vi "N-Parametric Double FFT Mesurament Test SLOW (con Sottrazione Fondo).vi"() -> ()   [LabVIEW 2014]
uses:
  <vilib>/Platform/TimedLoop/XDataNode/timing_clust.ctl
  <vilib>/Platform/TimedLoop/XDataNode/nitl_modes.ctl
  <vilib>/Platform/TimedLoop/XDataNode/wakeup.ctl
  <vilib>/rvi/Analysis/measure/FFT/simModelSupport/niFPGA FFT Streaming Sim Properties.ctl
  <vilib>/rvi/Analysis/measure/FFT/simModelSupport/niFPGA FFT Sim Stream Group Properties.ctl
  <vilib>/rvi/Analysis/measure/FFT/simModelSupport/niFPGA FFT Sim Types.ctl
  <vilib>/rvi/Analysis/measure/FFT/simModelSupport/niFpgaFFTSimArithmeticProperties.ctl
  <vilib>/rvi/Analysis/measure/FFT/simModelSupport/niFpgaFFTSimDfxp.ctl
  <vilib>/fxp/LVFixedPointQuantizationPolicyTypeDef.ctl
  <vilib>/rvi/Analysis/measure/FFT/XNode/niFpgaFFTButterflyDelays.ctl
  <vilib>/rvi/Emulation/niFpgaSctlEmulationGetInTimedLoop.vi
  <vilib>/rvi/Emulation/niFpgaEmulationReportErrorSimple.vi
  <vilib>/rvi/Emulation/niFpgaGetClockAttributes.vi
  <vilib>/rvi/Emulation/niFpgaCriticalErrorInLSC.vi
  <vilib>/rvi/Emulation/niFpgaEmulationIsFPGAContextNoSignature.vi
  <vilib>/rvi/DataTransferAndStorage/Container/Common/niFpgaContainerGetUniqueNameForEmu.vi
  <vilib>/rvi/Memory/Memory_Emulation/niFpgaMemoryEmulationCacheClearOnFirstRun.vi
  <vilib>/rvi/Memory/Memory_Emulation/nirvimemoryEmulationManagerCache_MakeExclusive.vi
  <vilib>/rvi/Memory/Memory_Emulation/niFpgaMemoryEmulationValidateCache.vi
  <vilib>/rvi/Memory/Memory_Emulation/nirvimemoryEmulationManagerCache_InsertValue.vi
  <vilib>/Utility/error.llb/Clear Errors.vi
  <vilib>/rvi/Memory/Memory_Emulation/nirvimemoryEmulationManagerCache_ReleaseExclusive.vi
  <vilib>/rvi/Memory/Memory_Emulation/nirvimemoryEmulationManagerCache_GetValue.vi
  <vilib>/rvi/Memory/Memory_Emulation/nirvimemoryEmulationManagerCache_SetValue.vi
  <vilib>/rvi/Emulation/niFpgaProcessEmulError.vi
  <vilib>/rvi/errors/niFpgaSetErrorForExecOnDevCompSimple.vi
  <vilib>/rvi/eio/common/nirviEmuReportErrorAndStop.vi
  <vilib>/rvi/FIFO/Fifo_Resource/nirvififoEmulationSetSize.vi
  <vilib>/rvi/FIFO/Fifo_Resource/nirviFifoEmulationQueueMgr.vi
  <instcachedir>/0/nirviFifoEmulationQueueMgr_E5CAEC123FF24DC58D834DCA3CDAA9B5.lvgen/nirviFifoEmulationQueueMgr_E5CAEC123FF24DC58D834DCA3CDAA9B5_010.vi
  <vilib>/rvi/FIFO/Fifo_Resource/nirvififoEmulationCreateLock.vi
  <vilib>/rvi/FIFO/Fifo_Resource/nirvififoEmulationObtainLock.vi
  <vilib>/rvi/FIFO/Fifo_Resource/nirvififoEmulationReleaseLock.vi
  <vilib>/rvi/occurrence/nirviWaitOnOccurrenceBase.vi
  <vilib>/rvi/errors/nirviReportUnexpectedCaseInternalError.vi
  <vilib>/rvi/errors/nirviReportUnexpectedCaseInternalError (U32).vi
  <vilib>/rvi/FIFO/Fifo_Resource/nirvififoEmulationDetermineInputValidOut.vi
  <vilib>/rvi/Memory/Memory_Emulation/nirvimemoryFastEmulation.vi
  <vilib>/rvi/Memory/Memory_Emulation/nirvimemoryEmulation.vi
  <vilib>/rvi/eio/common/nirviEmuTemplateMethod_errors.vi
  <vilib>/rvi/Analysis/measure/FFT/simModelSupport/niFpgaFFTSimModelStreamingCore.vi
  <vilib>/rvi/interface/RandomDataEmulation/niFpgaRandomDataHandleErrors.vi
  <vilib>/Platform/TimedLoop/XDataNode/XDataNode.xnode
  <vilib>/rvi/DataTransferAndStorage/Container/XNode/niFpgaContainer.xnode
  <vilib>/rvi/DataTransferAndStorage/Register/Emulation/niFpgaRegisterEmulation.vi
  <vilib>/rvi/FIFO/Fifo_Resource/nirvififoEmulationRead.vi
  <vilib>/rvi/FIFO/Fifo_Resource/nirvififoEmulationWrite.vi
  <vilib>/eio/EIOMethodNode/EIOMethodNode.xnode
  <vilib>/rvi/Analysis/measure/FFT/XNode/niFpgaFFT.xnode
  <vilib>/rvi/interface/RandomDataEmulation/nirviRandomDataFpgaReadWriteTemplate.vi
  <vilib>/Platform/TimedLoop/XDataNode/XDNodeRunTimeDep.lvlib
panel:
  in  "n-bit (2^nbit medie)":i32=8
  in  "n":u32=1
  in  "Latency points":u32
  in  "snapshot":bool
  in  "lower limit 2":u32=682
  in  "lower limit 1":u32=57
  in  "upper limit 2":u32=1193
  in  "upper limit 1":u32=568
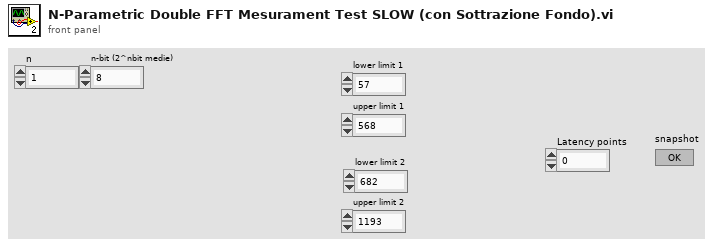
[diagram p1: front panel]
types:
  T1 = typedef "XDNodeRunTimeDep.lvlib/timing_clust.ctl" = cluster{"Expected End [f-1]":u64, "Actual End [f-1]":u64, "Finished Late? [f-1]":bool, "Expected End [i-1]":u64, "Actual End [i-1]":u64, "Finished Late? [i-1]":bool, "Expected Start [i]":u64, "Actual Start [i]":u64, "Expected Start [f]":u64, "Actual Start [f]":u64, "Source Name":string, "Structure Name":string, "Period":i64, "Deadline":i64, "Offset":i64, "Start":i64, "Priority":i32, "Timeout":i32, "Mode":T2, "Wakeup Reason":T3, "Error":errorcluster, "Source Type":string, "Secondary Source Type":string, "Global End Time":u64, "Global Start Time":u64, "Frame Duration":u64, "Iteration Duration":u64, "Assigned CPU":i32, "I/O Scan Engine Mode":u32}
  T2 = typedef "XDNodeRunTimeDep.lvlib/nitl_modes.ctl" = enum32{"No Change", "Process missed periods, maintain original phase", "Discard missed periods, maintain original phase", "Process missed periods, ignore original phase", "Discard missed periods, ignore original phase"}
  T3 = typedef "XDNodeRunTimeDep.lvlib/wakeup.ctl" = enum32{"Normal", "Aborted", "Asynchronous wakeup", "Timing source error", "Timed loop error", "Timeout"}
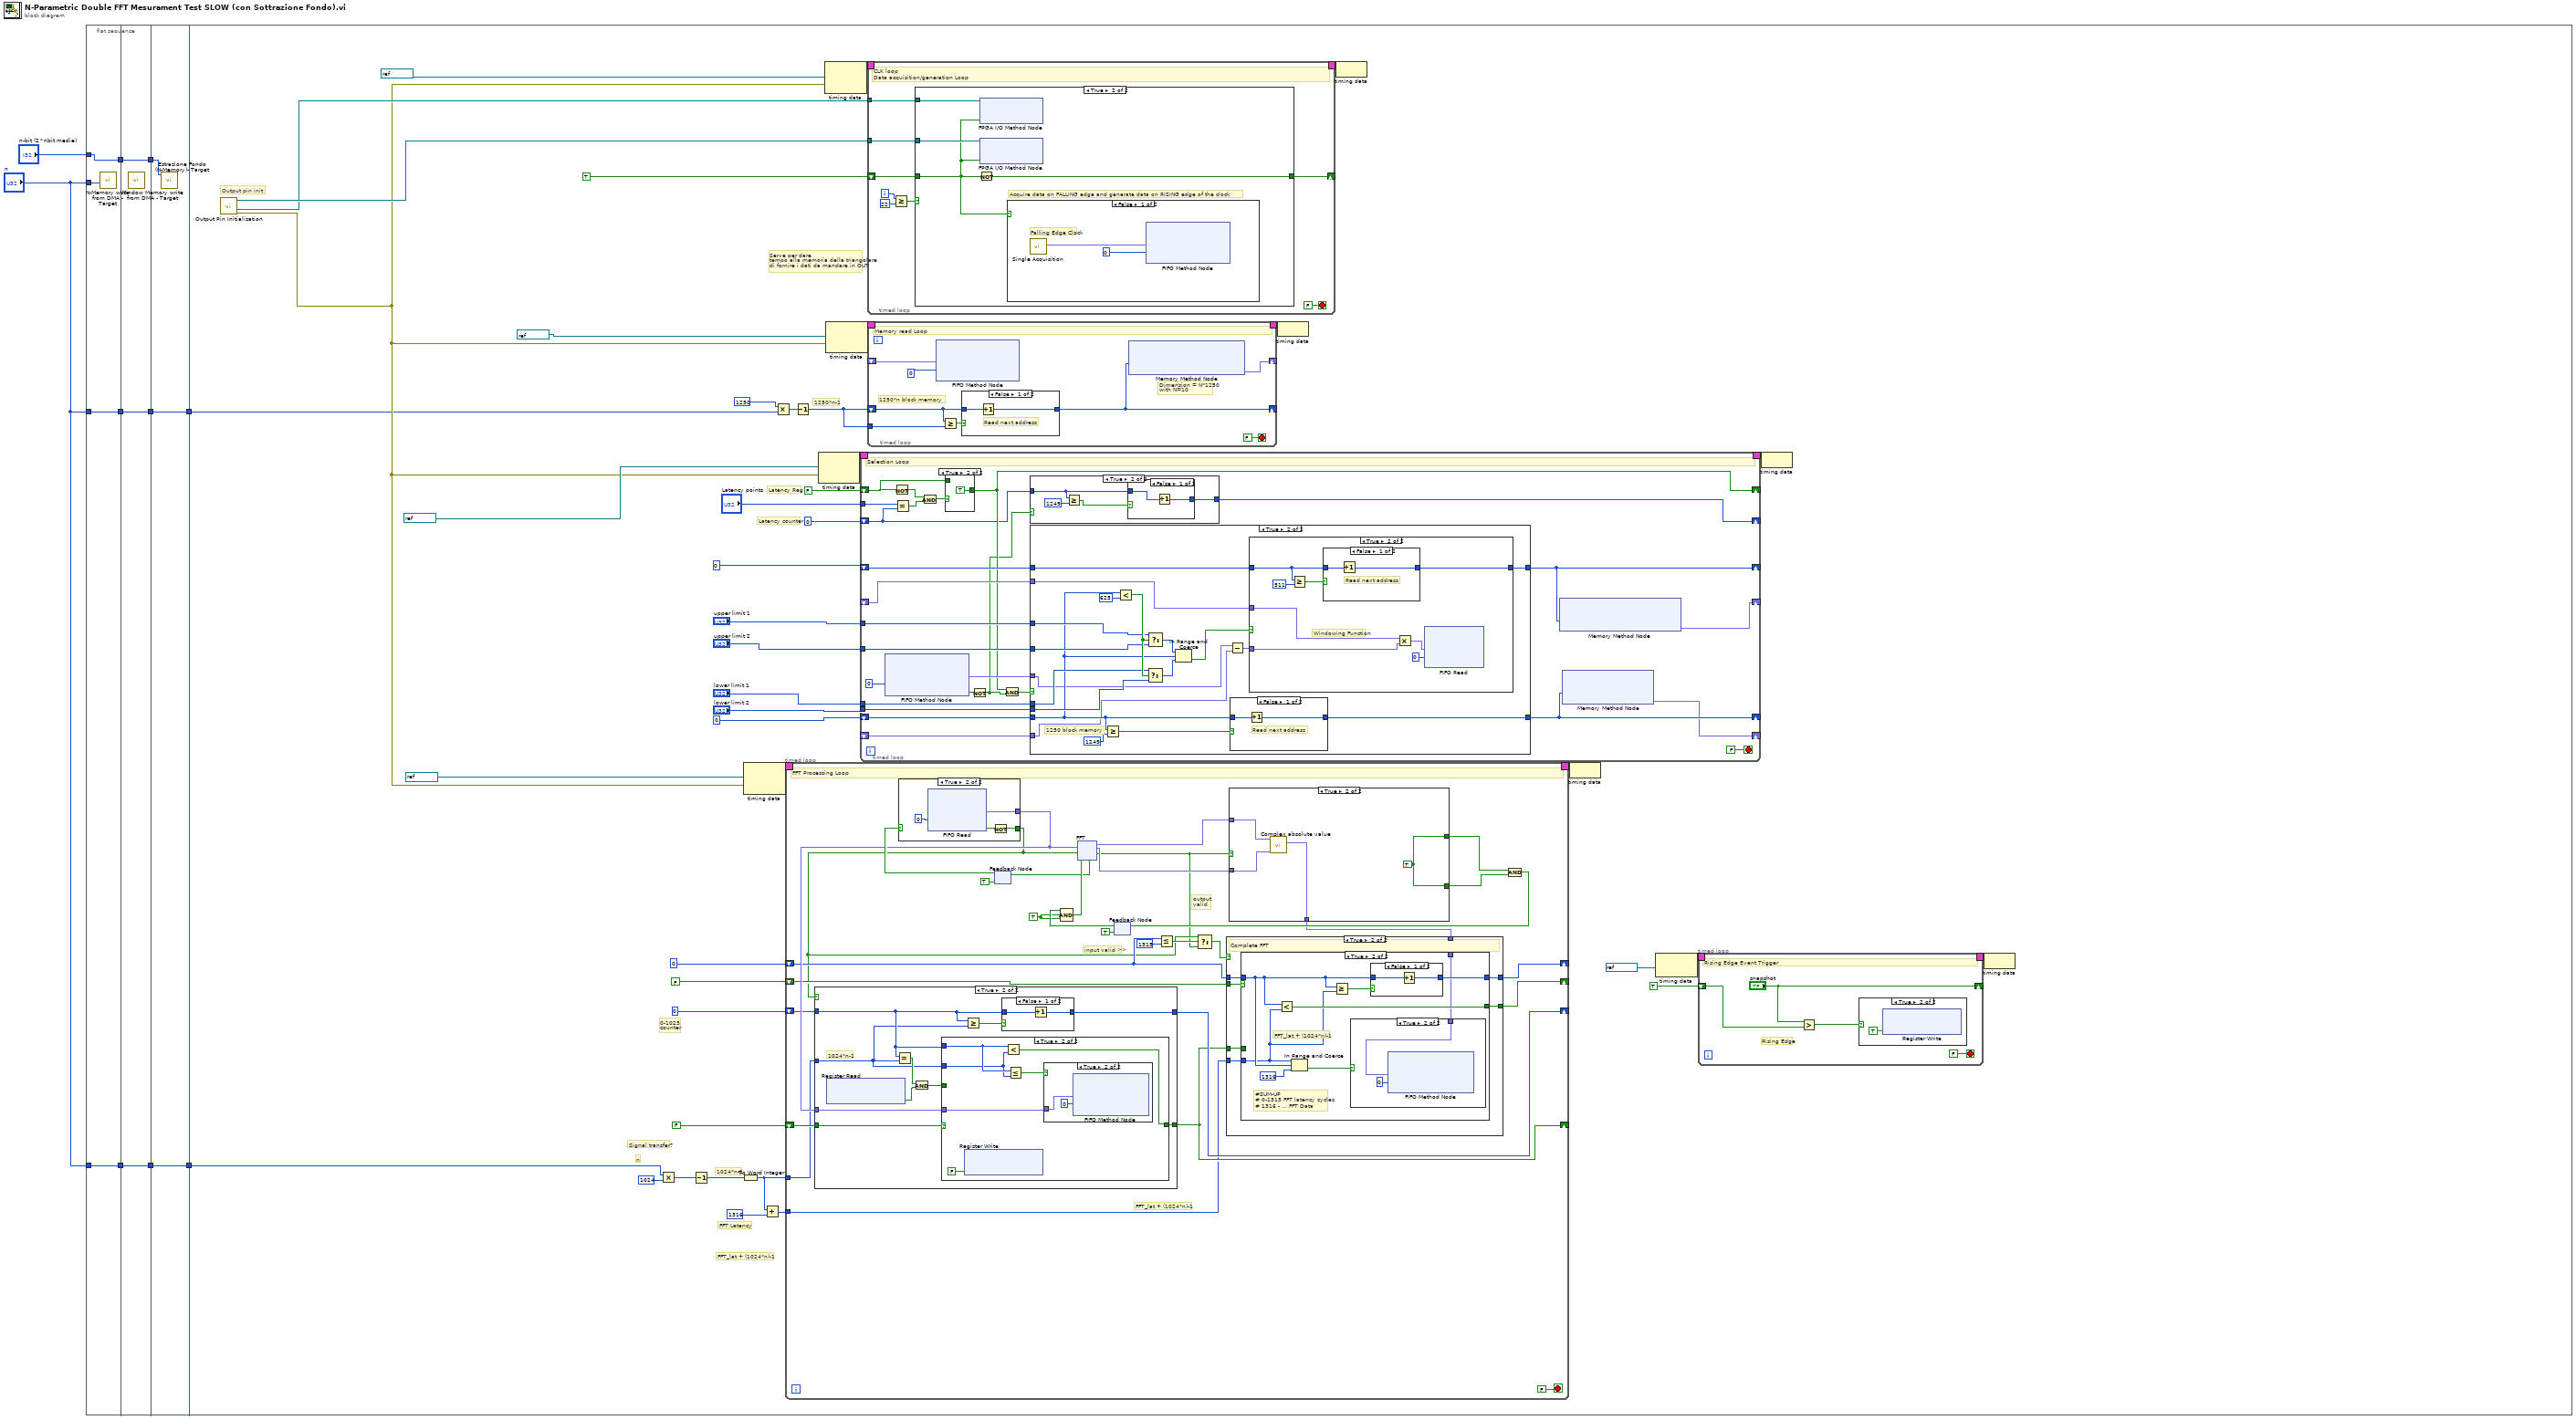
[diagram p0: block diagram]
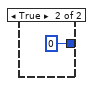
[diagram p4: hidden frame]
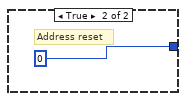
[diagram p8: hidden frame]
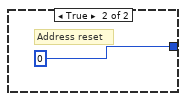
[diagram p9: hidden frame]
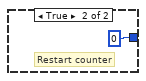
[diagram p13: hidden frame]
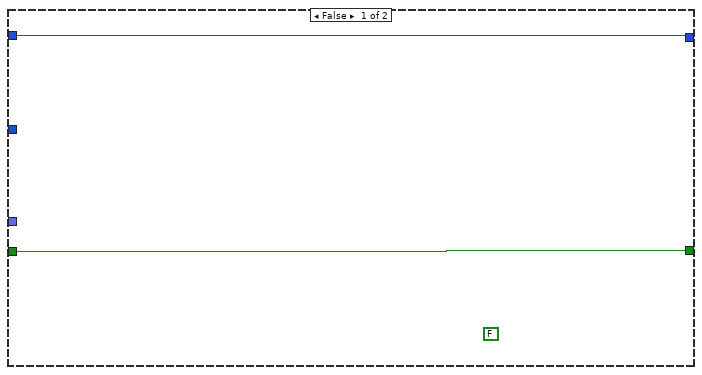
[diagram p14: hidden frame]
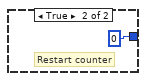
[diagram p17: hidden frame]
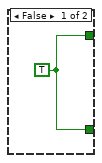
[diagram p18: hidden frame]
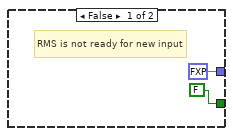
[diagram p19: hidden frame]
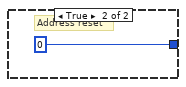
[diagram p20: hidden frame]
diagram:
  n1 = flat-sequence {
    tunnel: "n" -> [w14]
    tunnel: [w13] -> w10
    tunnel: "n" -> [w13]
    tunnel: "n" -> [w12]
    tunnel: [w12] -> w8
    tunnel: [w11] -> w3
    tunnel: "n-bit (2^nbit medie)" -> [w11]
    tunnel: w10 -> [w17]
    tunnel: [w17] -> w7
    tunnel: w8 -> [w16]
    tunnel: [w16] -> w5
    tunnel: w3 -> [w15]
    tunnel: [w15] -> w2
    tunnel: w7 -> [w20]
    tunnel: [w20] -> w6
    tunnel: w5 -> [w19]
    tunnel: [w19] -> w4
    tunnel: w2 -> [w18]
    tunnel: w6 -> [w30]
    tunnel: w4 -> [w21]
    frame #0 {
      n2 = call "N-Memory write from DMA - Target.vi"("n"=w14) -> ()  [unwired: 11 in]
    }
    frame #1 {
      n3 = call "Window Memory write from DMA - Target.vi"() -> ()  [unwired: 12 in]
    }
    frame #2 {
      n4 = call "Estrazione Fondo (N-Memory)- Target.vi"("n-bit (2^nbit medie)"=w18) -> ()  [unwired: 11 in]
    }
    frame #3 {
      # "1250*n-1"
      # "FFT_lat + (1024*n)-1"
      # "FFT Latency"
      # "n"
      # "1024*n-1"
      # "Serve per dare\ntempo alla memoria della triangolare\ndi fornire i dati da mandare in OUT"
      # "Latency counter"
      # "Latency Reg"
      # "0-1023\ncounter"
      # "Signal transfer?"
      # "Output pin init"
      n5 = call "Output Pin Initialization.vi"() -> ("error out"=w48:errorcluster, "I/O Out Clock DAC (pin16)"=w52:refnum<k21>, "I/O Out Clock ADC (pin17)"=w53:refnum<k21>)  [unwired: 8 in]
      n6 = Multiply(x=w30, y=u32 1024) -> (x*y=w31:u32)
      n7 = Decrement(x=w31) -> (x-1=w29:u32)
      n8 = To Word Integer(number=w29) -> (16bit integer=w27:i16)
      n9 = node-c288(refnum<k21> "30MHz" ("Source Name"), w48) -> (w60:T1)
      n10 = Add(x=w27, y=i16 1316) -> (x+y=w25:i16)
      n11 = Multiply(x=u32 1250, y=w21) -> (x*y=w23:u32)
      n12 = timed-loop {
        timing: w60 -> [_]
        timing-out: [_] -> w59
        shift-right: [w168] -> _
        shift-left: FALSE -> [w171]
        shift-right: [w172] -> _
        shift-left: i16 0 -> [w169]
        shift-right: [w167] -> _
        shift-left: FALSE -> [w166]
        shift-right: [w165] -> _
        shift-left: i16 0 -> [w163]
        tunnel: w27 -> [w156]
        tunnel: w25 -> [w155]
        stop <- FALSE stop-if-true
        w157 = TRUE
        # "FFT_lat + (1024*n)-1"
        # "output\nvalid"
        # "input valid >>"
        # "FFT Processing Loop"
        n13 = feedback #1(TRUE ("ready for input")) -> (w184:bool)
        n14 = case shown="True" w184 {
          tunnel: [FALSE w269] -> w159
          tunnel: [fxp<+/-,12,12> 0.0 ("Element") w266] -> w170
          frame False {
            # "RMS is not ready for new input"
          }
          frame True {
            n15 = xnode ("FIFO Read")("Timeout"=0) -> ("Element"=w266:fxp<+/-,12,12>, "Timed Out?"=w268:bool)  [unwired: 1 in, 1 out]
            n16 = Not(x=w268) -> (.not. x?=w269:bool)
          }
        }
        n17 = case shown="True" w159 {
          tunnel: w169 -> [w210 w216]
          tunnel: [w210 w219] -> w172
          tunnel: w171 -> [w209 w214]
          tunnel: [w209 w215] -> w168
          tunnel: w170 -> [_ w213]
          tunnel: w156 -> [_ w211]
          frame False {
            (unwired) FALSE
          }
          frame True {
            # "1024*n-1"
            n18 = xnode ("Register Read")() -> ("Data"=w212:bool)  [unwired: 1 in, 1 out]
            n19 = Equal?(x=w216, y=w211) -> (x = y?=w218:bool)
            n20 = And(x=w218, y=w212) -> (x .and. y?=w217:bool)
            n21 = case shown="True" w214 {
              tunnel: w217 -> [w221 _]
              tunnel: w216 -> [_ w223]
              tunnel: [w221 w227] -> w215
              tunnel: w213 -> [_ w225]
              tunnel: w211 -> [_ w222]
              frame False {
              }
              frame True {
                n22 = xnode ("Register Write")("Data"=FALSE) -> ()  [unwired: 1 in, 1 out]
                n23 = Less?(x=w223, y=w222) -> (x < y?=w227:bool)
                n24 = Less Or Equal?(x=w223, y=w222) -> (x <= y?=w226:bool)
                n25 = case shown="True" w226 {
                  tunnel: w225 -> [_ w228]
                  frame False {
                  }
                  frame True {
                    n26 = xnode ("FIFO Method Node")("Element"=w228, "Timeout"=0) -> ()  [unwired: 1 in, 2 out]
                  }
                }
              }
            }
            n27 = Greater Or Equal?(x=w216, y=w211) -> (x >= y?=w220:bool)
            n28 = case shown="False" w220 {
              tunnel: w216 -> [w231 _]
              tunnel: [w230 i16 0] -> w219
              frame False {
                n29 = Increment(x=w231) -> (x+1=w230:i16)
              }
              frame True {
                # "Restart counter"
              }
            }
          }
        }
        n30 = feedback #2(TRUE) -> (w180:bool)
        n31 = Compound Arithmetic op=AND(w180, w157, w157) -> (w179:bool)
        n32 = xnode "FFT"("real data in"=w170, "input valid"=w159, "ready for output"=w179) -> ("ready for input"=w178:bool, "real data out"=w177:fxp<+/-,22,22>, "imaginary data out"=w176:fxp<+/-,22,22>, "output valid"=w158:bool)  [unwired: 2 in, 1 out]
        n33 = feedback-in #1(w178) -> ()
        n34 = Less Or Equal?(x=w163, y=i16 1315) -> (x <= y?=w164:bool)
        n35 = Select(t=w159, s=w164, f=w158) -> (s? t:f=w161:bool)
        n36 = case shown="True" w158 {
          tunnel: w177 -> [_ w263]
          tunnel: w176 -> [_ w262]
          tunnel: [w259 w260] -> w175
          tunnel: [w259 w260] -> w174
          tunnel: [_ w261] -> w160
          frame False {
            w259 = TRUE
          }
          frame True {
            w260 = TRUE
            n37 = call "Complex absolute value.vi"("Im"=w262, "Re"=w263) -> ("Square Absolute Value"=w261:fxp<+,44,44>)  [unwired: 9 in]
          }
        }
        n38 = case shown="True" w161 {
          tunnel: w168 -> [_ w193]
          tunnel: [w185 w192] -> w167
          tunnel: w166 -> [w185 w191]
          tunnel: w163 -> [w186 w190]
          tunnel: [w186 w189] -> w165
          tunnel: w160 -> [_ w188]
          tunnel: w155 -> [_ w187]
          frame False {
          }
          frame True {
            # "Complete FFT"
            n39 = case shown="True" w191 {
              tunnel: w193 -> [w195 _]
              tunnel: [w195 w203] -> w192
              tunnel: w190 -> [w194 w199]
              tunnel: [w194 w201] -> w189
              tunnel: w188 -> [_ w197]
              tunnel: w187 -> [_ w196]
              frame False {
              }
              frame True {
                # "FFT_lat + (1024*n)-1"
                # "#SUM-UP\n# 0-1315 FFT latency cycles\n# 1316 - ... FFT Data"
                n40 = Less?(x=w199, y=w196) -> (x < y?=w203:bool)
                n41 = In Range and Coerce(upper limit=w196, x=w199, lower limit=i16 1316 ("y")) -> (In Range?=w198:bool)  [unwired: 1 out]
                n42 = Greater Or Equal?(x=w199, y=w196) -> (x >= y?=w202:bool)
                n43 = case shown="True" w198 {
                  tunnel: w197 -> [_ w205]
                  frame False {
                  }
                  frame True {
                    n44 = xnode ("FIFO Method Node")("Element"=w205, "Timeout"=0) -> ()  [unwired: 1 in, 2 out]
                  }
                }
                n45 = case shown="False" w202 {
                  tunnel: w199 -> [w207 _]
                  tunnel: [w206 i16 0] -> w201
                  frame False {
                    n46 = Increment(x=w207) -> (x+1=w206:i16)
                  }
                  frame True {
                    # "Restart counter"
                  }
                }
              }
            }
          }
        }
        n47 = Compound Arithmetic op=AND(w175, w174) -> (w173:bool)
        n48 = feedback-in #2(w173) -> ()
      }
      n49 = Decrement(x=w23) -> (x-1=w22:u32)
      n50 = node-c288(refnum<k21> "30MHz" ("Source Name"), w48) -> (w58:T1)
      n51 = node-c288(refnum<k21> "60MHz" ("Source Name"), w48) -> (w64:T1)
      n52 = node-c288(refnum<k21> "30MHz" ("Source Name"), w48) -> (w62:T1)
      n53 = timed-loop {
        timing: w58 -> [_]
        timing-out: [_] -> w57
        shift-right: [w77] -> _
        shift-left: u32 0 -> [w88]
        tunnel: "upper limit 1" -> [w97]
        tunnel: "upper limit 2" -> [w96]
        tunnel: "lower limit 1" -> [w95]
        tunnel: "lower limit 2" -> [w94]
        shift-right: [w90] -> _
        shift-left: u32 0 -> [w93]
        shift-right: [w91] -> _
        shift-left: _ -> [w92]
        shift-right: [w82] -> _
        shift-left: FALSE -> [w83]
        tunnel: "Latency points" -> [w87]
        shift-right: [w80] -> _
        shift-left: u32 0 -> [w79]
        shift-right: [w76] -> _
        shift-left: _ -> [w78]
        stop <- FALSE stop-if-true
        # "Selection Loop"
        n54 = xnode ("FIFO Method Node")("Timeout"=0) -> ("Element"=w99:fxp<+/-,12,12>, "Timed Out?"=w100:bool)  [unwired: 1 in, 1 out]
        n55 = Not(x=w83) -> (.not. x?=w86:bool)
        n56 = Equal?(x=w87, y=w79) -> (x = y?=w85:bool)
        n57 = And(x=w86, y=w85) -> (x .and. y?=w84:bool)
        n58 = case shown="True" w84 {
          tunnel: [w110 TRUE] -> w82
          tunnel: w83 -> [w110 _]
          frame False {
          }
          frame True {
          }
        }
        n59 = Not(x=w100) -> (.not. x?=w81:bool)
        n60 = And(x=w82, y=w81) -> (x .and. y?=w89:bool)
        n61 = case shown="True" w81 {
          tunnel: w79 -> [w102 w105]
          tunnel: [w102 w103] -> w80
          frame False {
          }
          frame True {
            n62 = Greater Or Equal?(x=w105, y=u32 1249) -> (x >= y?=w104:bool)
            n63 = case shown="False" w104 {
              tunnel: w105 -> [w108 _]
              tunnel: [w107 u32 0] -> w103
              frame False {
                n64 = Increment(x=w108) -> (x+1=w107:u32)
              }
              frame True {
              }
            }
          }
        }
        n65 = case shown="True" w89 {
          tunnel: [w113 w130] -> w77
          tunnel: w88 -> [w113 w118]
          tunnel: w99 -> [_ w115]
          tunnel: w97 -> [_ w125]
          tunnel: w96 -> [_ w124]
          tunnel: w95 -> [_ w123]
          tunnel: w94 -> [_ w122]
          tunnel: w93 -> [w112 w119]
          tunnel: [w112 w121] -> w90
          tunnel: w92 -> [_ w120]
          tunnel: w78 -> [_ w114]
          frame False {
          }
          frame True {
            # "1250 block memory"
            n66 = Greater Or Equal?(x=w118, y=u32 1249) -> (x >= y?=w131:bool)
            n67 = Less?(x=w118, y=u32 625) -> (x < y?=w126:bool)
            n68 = Select(t=w123, s=w126, f=w122) -> (s? t:f=w128:u32)
            n69 = Select(t=w125, s=w126, f=w124) -> (s? t:f=w129:u32)
            n70 = In Range and Coerce(upper limit=w129, x=w118, lower limit=w128) -> (In Range?=w117:bool)  [unwired: 1 out]
            n71 = Subtract(x=w115, y=w114) -> (x-y=w116:fxp<+/-,12,12>)
            n72 = case shown="False" w131 {
              tunnel: w118 -> [w146 _]
              tunnel: [w145 u32 0] -> w130
              frame False {
                # "Read next address"
                n73 = Increment(x=w146) -> (x+1=w145:u32)
              }
              frame True {
                # "Address reset"
              }
            }
            n74 = case shown="True" w117 {
              tunnel: w116 -> [_ w134]
              tunnel: w119 -> [w133 w139]
              tunnel: [w133 w141] -> w121
              tunnel: w120 -> [_ w137]
              frame False {
              }
              frame True {
                # "Windowing Function"
                n75 = Greater Or Equal?(x=w139, y=u32 511) -> (x >= y?=w140:bool)
                n76 = case shown="False" w140 {
                  tunnel: w139 -> [w143 _]
                  tunnel: [w142 u32 0] -> w141
                  frame False {
                    # "Read next address"
                    n77 = Increment(x=w143) -> (x+1=w142:u32)
                  }
                  frame True {
                    # "Address reset"
                  }
                }
                n78 = Multiply(x=w137, y=w134) -> (x*y=w135:fxp<+/-,12,12>)
                n79 = xnode ("FIFO Read")("Element"=w135, "Timeout"=0) -> ()  [unwired: 1 in, 2 out]
              }
            }
          }
        }
        n80 = xnode ("Memory Method Node")("Address"=w90) -> ("Data"=w91:fxp<+,8,1>)  [unwired: 1 in, 1 out]
        n81 = xnode ("Memory Method Node")("Address"=w77) -> ("Data"=w76:fxp<+/-,12,12>)  [unwired: 1 in, 1 out]
      }
      n82 = timed-loop {
        timing: w64 -> [_]
        timing-out: [_] -> w63
        shift-right: [w300] -> _
        shift-left: TRUE -> [w298]
        tunnel: w52 -> [w302]
        tunnel: w53 -> [w299]
        i -> [w296]
        stop <- FALSE stop-if-true
        # "CLK loop\nData acquisition/generation Loop"
        n83 = Greater Or Equal?(x=w296, y=22) -> (x >= y?=w295:bool)
        n84 = case shown="True" w295 {
          tunnel: w302 -> [_ w307]
          tunnel: [w303 w306] -> w300
          tunnel: w299 -> [_ w305]
          tunnel: w298 -> [w303 w304]
          frame False {
          }
          frame True {
            # "Acquire data on FALLING edge and generate data on RISING edge of the clock"
            n85 = Not(x=w304) -> (.not. x?=w306:bool)
            n86 = xnode "FPGA I/O Method Node"("FPGA I/O In"=w307, "Data"=w304) -> ()  [unwired: 1 out]
            n87 = xnode "FPGA I/O Method Node"("FPGA I/O In"=w305, "Data"=w304) -> ()  [unwired: 1 out]
            n88 = case shown="False" w304 {
              frame False {
                # "Falling Edge Clock"
                n89 = call "Single Acquisition.vi"() -> ("Out"=w309:fxp<+/-,12,12>)  [unwired: 10 in, 1 out]
                n90 = xnode ("FIFO Method Node")("Element"=w309, "Timeout"=0) -> ()  [unwired: 1 in, 2 out]
              }
              frame True {
                # "Rising Edge Clock"
                n91 = xnode ("FIFO Method Node")("Timeout"=0) -> ("Element"=w310:fxp<+/-,12,12>, "Timed Out?"=w311:bool)  [unwired: 1 in, 1 out]
                n92 = case shown="False" w311 {
                  tunnel: w310 -> [w315 _]
                  frame False {
                    # "Data Generation"
                    n93 = Add(x=w315, y=fxp<+,12,12> 2048.0) -> (x+y=w313:fxp<+/-,14,14>)
                    n94 = call "Single Point Wave generation.vi"("Data To Write"=w313) -> ()  [unwired: 10 in, 1 out]
                  }
                  frame True {
                    # "FPGA memory slow"
                  }
                }
              }
            }
          }
        }
      }
      n95 = timed-loop {
        timing: w62 -> [_]
        timing-out: [_] -> w61
        shift-right: [w278] -> _
        shift-left: w22 -> [w282]
        shift-right: [w280] -> _
        shift-left: _ -> [w279]
        tunnel: w22 -> [w277]
        stop <- FALSE stop-if-true
        # "Dimension = N*1250\nwith N=10"
        # "1250*n block memory"
        # "Memory read Loop"
        n96 = xnode ("FIFO Method Node")("Element"=w279, "Timeout"=0) -> ()  [unwired: 1 in, 2 out]
        n97 = Greater Or Equal?(x=w282, y=w277) -> (x >= y?=w284:bool)
        n98 = case shown="False" w284 {
          tunnel: w282 -> [w286 _]
          tunnel: [w285 u32 0] -> w278
          frame False {
            # "Read next address"
            n99 = Increment(x=w286) -> (x+1=w285:u32)
          }
          frame True {
            # "Address reset"
          }
        }
        n100 = xnode ("Memory Method Node")("Address"=w278) -> ("Data"=w280:fxp<+/-,12,12>)  [unwired: 1 in, 1 out]
      }
      n101 = node-c288(w61) -> ()
      n102 = node-c288(w63) -> ()
      n103 = node-c288(w59) -> ()
      n104 = node-c288(refnum<k21> "30MHz" ("Source Name")) -> (w38:T1)
      n105 = timed-loop {
        timing: w38 -> [_]
        timing-out: [_] -> w37
        shift-right: ["snapshot"] -> _
        shift-left: TRUE ("snapshot") -> [w67]
        stop <- FALSE stop-if-true
        # "Rising Edge"
        # "Rising Edge Event Trigger"
        n106 = Greater?(x="snapshot", y=w67) -> (0:w65:bool)
        n107 = case shown="True" w65 {
          frame False {
          }
          frame True {
            n108 = xnode ("Register Write")("Data"=TRUE) -> ()  [unwired: 1 in, 1 out]
          }
        }
      }
      n109 = node-c288(w57) -> ()
      n110 = node-c288(w37) -> ()
    }
  }
